vi "Get Ctl Value.vi"(8 "error in (no error)":errorcluster, 11 "Text field in":refnum<class "Text field.lvclass">) -> (0 "error out":errorcluster, 2 "Value":string, 3 "Text field out":refnum<class "Text field.lvclass">)   [LabVIEW 2020, in "Basic Fields.lvlib" / "Text field.lvclass"]
uses:
  Text field.lvclass
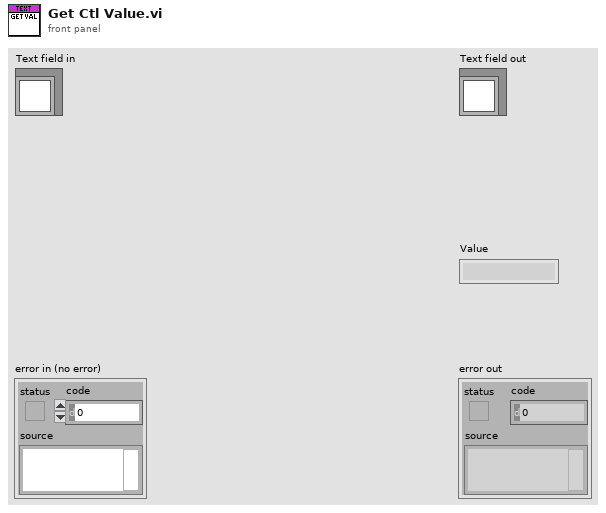
[diagram p1: front panel]
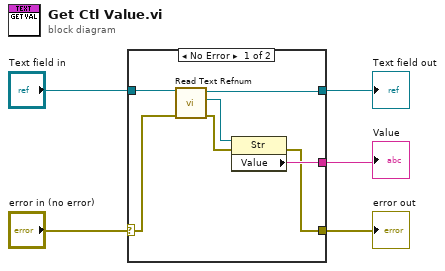
[diagram p0: block diagram]
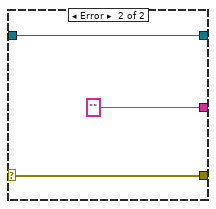
[diagram p2: hidden frame]
diagram:
  n1 = case shown="No Error" "error in (no error)" {
    selector: "error in (no error)" -> [w11 w14]
    tunnel: "Text field in" -> [w12 w15]
    tunnel: [w10 w15] -> w3
    tunnel: [w6 w14] -> w2
    tunnel: [w8 "" ("Value")] -> w1
    frame No Error {
      n2 = call "Read Text Refnum.vi"("error in (no error)"=w11, "Text field in"=w12) -> ("error out"=w7:errorcluster, "Str Refnum"=w9:refnum<vi>, "Text field out"=w10:refnum<class "Text field.lvclass">)  [unwired: 7 in]
      n3 = property class="Str"(reference=w9, error in=w7) -> (error out=w6:errorcluster, "Value"=w8:string)  [unwired: 1 out]
    }
    frame Error {
    }
  }
  "error out" <- w2
  "Text field out" <- w3
  "Value" <- w1
